vi "Test Semaphore 4.vi"() -> ()   [LabVIEW 2011]
panel:
  out "Iterations":i32
  in  "milliseconds to hold":u32=500
  in  "milliseconds to wait":u32=500
  out "Wait Time":u32
  out "Hold Time":u32
  out "millisecond timer value 1":u32
  out "Prior Count":i32
  out "millisecond timer value 2":u32
  out "Locked 1":bool
  out "Numeric":i32
  out "Timed Out? 1":bool
  out "error out rel 2":errorcluster
  out "error out acq 2":errorcluster
  in  "Acq":bool
  in  "Open":bool
  in  "stop":bool
  out "Handle":u16
  out "error out create":errorcluster
  in  "Name":string="LabVIEW_System_Semaphore"
  out "error out destroy 1":errorcluster
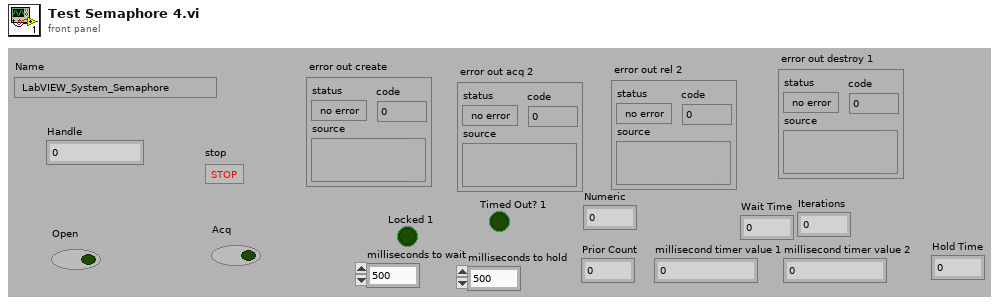
[diagram p1: front panel]
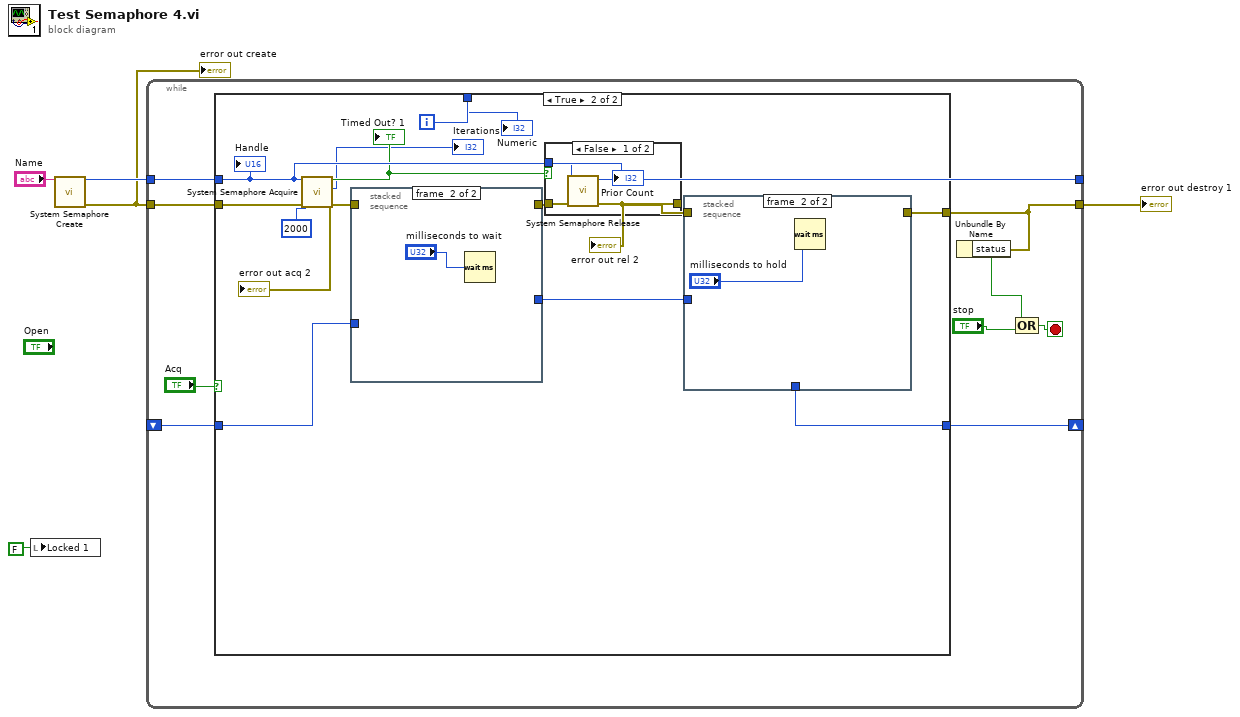
[diagram p0: block diagram]
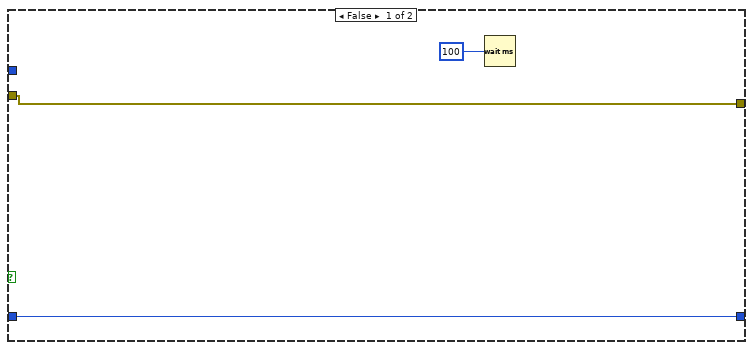
[diagram p2: hidden frame]
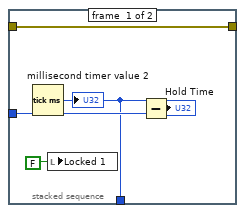
[diagram p4: hidden frame]
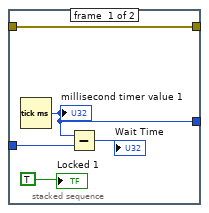
[diagram p5: hidden frame]
diagram:
  n1 = local write "Locked 1"(FALSE) -> ()
  n2 = call "System Semaphore Create.vi"("Name"="Name") -> ("error out"=w3:errorcluster, "Handle"=w5:u16)  [unwired: 9 in]
  "error out create" <- w3
  n3 = while {
    tunnel: w3 -> [w8]
    tunnel: w5 -> [w11]
    tunnel: [w11] -> _
    tunnel: [w10] -> w1
    shift-right: [w7] -> _
    shift-left: _ -> [w6]
    i -> [w12]
    stop <- w14 stop-if-true
    n4 = case shown="True" "Acq" {
      tunnel: w12 -> [_ w31]
      tunnel: w11 -> [_ w25]
      tunnel: [w18 w29] -> w10
      tunnel: w8 -> [w18 w24]
      tunnel: [w16 w22] -> w7
      tunnel: w6 -> [w16 w21]
      frame False {
        n5 = Wait (ms)(milliseconds to wait=u32 100) -> ()  [unwired: 1 out]
      }
      frame True {
        n6 = call "System Semaphore Acquire.vi"("error in (no error)"=w24, "Timeout (ms)"=u16 2000, "SemaphoreHandle"=w25) -> ("error out"=w28:errorcluster, "Iterations"=→"Iterations":i16, "Timed Out?"=w20:bool)  [unwired: 6 in]
        "Timed Out? 1" <- w20
        "error out acq 2" <- w28
        n7 = stacked-sequence {
          tunnel: w28 -> [w47 _]
          tunnel: [w47 _] -> w27
          tunnel: [w44 _] -> w23
          tunnel: w21 -> [w43 _]
          frame #0 {
            n8 = Tick Count (ms)() -> (millisecond timer value=w44:u32)
            "millisecond timer value 1" <- w44
            n9 = Subtract(x=w44, y=w43) -> (x-y=→"Wait Time":u32)
            "Locked 1" <- TRUE
          }
          frame #1 {
            n10 = Wait (ms)(milliseconds to wait="milliseconds to wait") -> ()  [unwired: 1 out]
          }
        }
        n11 = case shown="False" w20 {
          tunnel: w27 -> [w35 w36]
          tunnel: w25 -> [w34 _]
          tunnel: [w33 w36] -> w26
          frame False {
            n12 = call "System Semaphore Release.vi"("error in (no error)"=w35, "SemaphoreHandle"=w34) -> ("error out"=w33:errorcluster, "PreviousCount"=→"Prior Count":i32)  [unwired: 8 in]
          }
          frame True {
          }
        }
        "error out rel 2" <- w26
        n13 = stacked-sequence {
          tunnel: w26 -> [w41 _]
          tunnel: [w41 _] -> w29
          tunnel: w23 -> [w39 _]
          tunnel: [w37 _] -> w22
          frame #0 {
            n14 = Tick Count (ms)() -> (millisecond timer value=w37:u32)
            "millisecond timer value 2" <- w37
            n15 = local write "Locked 1"(FALSE) -> ()
            n16 = Subtract(x=w37, y=w39) -> (x-y=→"Hold Time":u32)
          }
          frame #1 {
            n17 = Wait (ms)(milliseconds to wait="milliseconds to hold") -> ()  [unwired: 1 out]
          }
        }
        "Handle" <- w25
        "Numeric" <- w31
      }
    }
    n18 = Unbundle By Name(w10) -> ("status"=w13:bool)
    n19 = Compound Arithmetic op=OR(w13, "stop") -> (w14:bool)
  }
  "error out destroy 1" <- w1
